vi "G#SubClass2_Create.vi"(0 "reference in":refnum<class "G#SubClass2.lvclass">, 1 "object name":string, 4 "no registration":bool, 5 "error in (no error)":errorcluster, 6 "create method":T1=enum."Create or look up existing", 7 "user counter":bool=TRUE) -> (14 "reference out":refnum<class "G#SubClass2.lvclass">, 19 "error out":errorcluster)   [LabVIEW 2017, in "G#SubClass2.lvclass"]
doc: "Constructor."
uses:
  G#SubClass2.lvclass
  C:/Program Files/National Instruments/LabVIEW 2017/vi.lib/addons/_AddQ/G#Object/G#Object.lvclass
  C:/Projects/GsharpGIT2017/Verification/TestCases/TestClasses/G#BaseClass2_class/G#BaseClass2.lvclass
  <vilib>/addons/_AddQ/G#Object/utils/G#Object_CreateMethod.ctl
  <vilib>/addons/_AddQ/G#Object/G#Object.lvclass
  G#BaseClass2_class/G#BaseClass2.lvclass
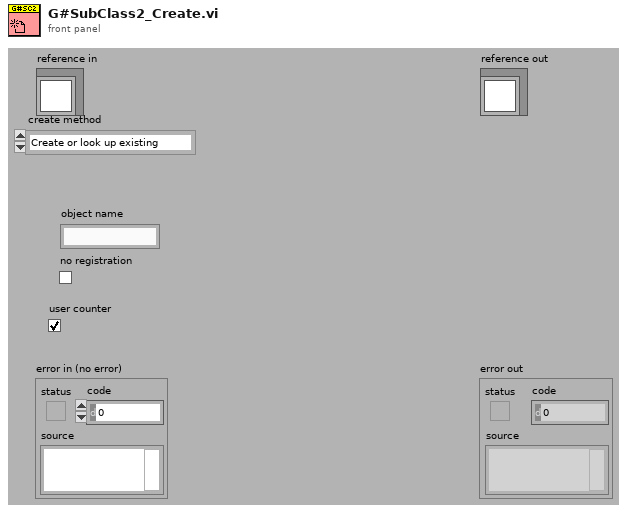
[diagram p1: front panel]
types:
  T1 = typedef "G#Object.lvclass/G#Object_CreateMethod.ctl" = enum16{"Create", "Create or look up existing", "Look up existing"}
  T2 = typedef "G#SubClass2.lvclass/ObjectAttributes.ctl" = cluster{"Base class":T3, "SubAttribute":dbl}
  T3 = typedef "G#BaseClass2.lvclass/ObjectAttributes.ctl" = cluster{"Numeric":dbl, "Array":dbl[]}
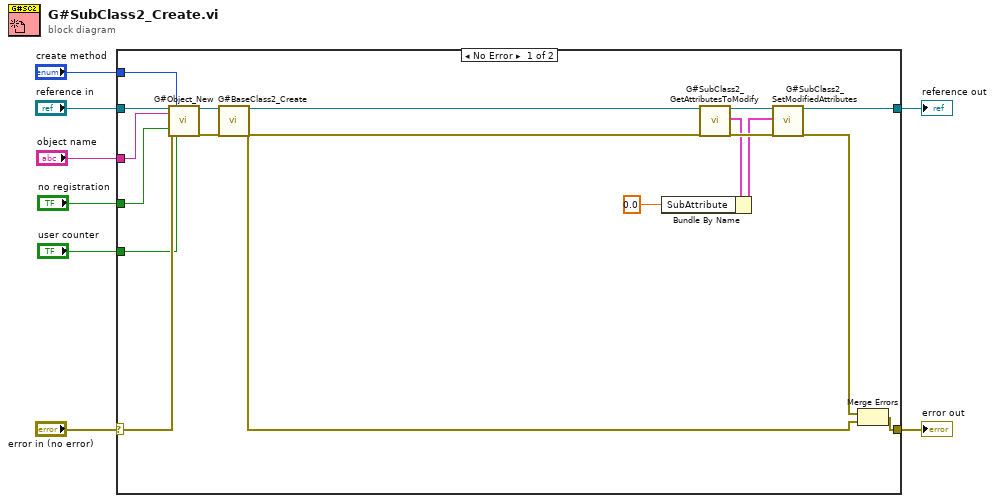
[diagram p0: block diagram]
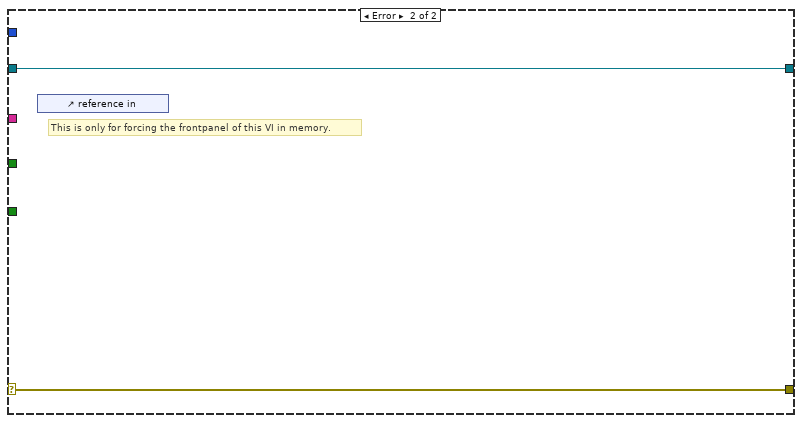
[diagram p2: hidden frame]
diagram:
  n1 = case shown="No Error" "error in (no error)" {
    selector: "error in (no error)" -> [w25 w28]
    tunnel: [w24 w28] -> w7
    tunnel: [w19 w27] -> w5
    tunnel: "reference in" -> [w26 w27]
    tunnel: "create method" -> [w12 _]
    tunnel: "object name" -> [w11 _]
    tunnel: "no registration" -> [w10 _]
    tunnel: "user counter" -> [w9 _]
    frame No Error {
      n2 = call <vilib>:"G#Object_New.vi"("reference in"=w26, "object name"=w11, "no registration? (F)"=w10, "error in (no error)"=w25, "create method"=w12, "user counter (T)?"=w9) -> ("reference out"=w23:refnum<class "G#SubClass2.lvclass">, "error out"=w22:errorcluster)  [unwired: 11 in, 1 out]
      n3 = call "G#BaseClass2_Create.vi"("reference in"=w23, "error in (no error)"=w22) -> ("reference out"=w20:refnum<class "G#SubClass2.lvclass">, "error out"=w18:errorcluster)  [unwired: 16 in]
      n4 = call "G#SubClass2_GetAttributesToModify.vi"("reference in"=w20, "error in (no error)"=w18) -> ("reference out"=w21:refnum<class "G#SubClass2.lvclass">, "attributes"=w15:T2, "error out"=w17:errorcluster)  [unwired: 13 in, 2 out]
      n5 = Bundle By Name(cluster=w15, "SubAttribute"=0.0 ("Base class.Numeric")) -> (w14:T2)
      n6 = call "G#SubClass2_SetModifiedAttributes.vi"("reference in"=w21, "attributes"=w14, "error in (no error)"=w17) -> ("reference out"=w19:refnum<class "G#SubClass2.lvclass">, "error out"=w16:errorcluster)  [unwired: 15 in]
      n7 = Merge Errors(w16, w18) -> (w24:errorcluster)
    }
    frame Error {
      # "This is only for forcing the frontpanel of this VI in memory."
      n8 = control-ref of="reference in"() -> ()  [unwired: 1 out]
    }
  }
  "error out" <- w7
  "reference out" <- w5
